vi "ConvertVoltToDegree.vi"(10 "Tension":dbl) -> (2 "Température":dbl)   [LabVIEW 2018]
panel:
  out "x+y":dbl
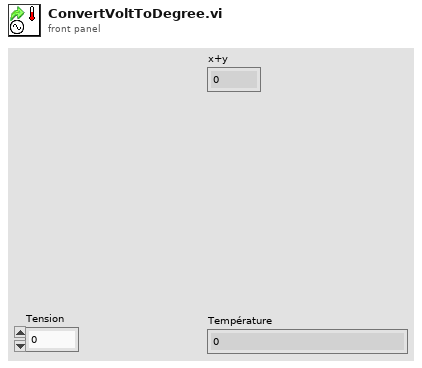
[diagram p1: front panel]
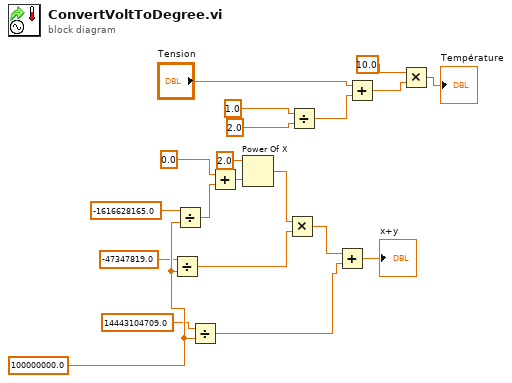
[diagram p0: block diagram]
diagram:
  w16 = 100000000.0
  n1 = Divide(x=-47347819.0, y=w16) -> (x/y=w19:dbl)
  n2 = Divide(x=-1616628165.0, y=w16) -> (x/y=w20:dbl)
  n3 = Divide(x=14443104709.0, y=w16) -> (x/y=w18:dbl)
  n4 = Add(x=0.0, y=w20) -> (x+y=w12:dbl)
  n5 = Power Of X(1:w12, 2:2.0 ("y")) -> (0:w11:dbl)
  n6 = Multiply(x=w11, y=w19) -> (x*y=w17:dbl)
  n7 = Divide(x=1.0, y=2.0) -> (x/y=w5:dbl)
  n8 = Add(x=w17, y=w18) -> (x+y=→"x+y":dbl)
  n9 = Add(x="Tension", y=w5) -> (x+y=w3:dbl)
  n10 = Multiply(x=10.0, y=w3) -> (x*y=→"Température":dbl)
